vi "Initialize.vi"(5 "plugin settings":T1[](array[typedef]), 7 "Components":refnum<class "Component.lvclass">[](array[class]), 8 "error in (no error)":errorcluster, 9 "Group Configurations":refnum<class "Group Configuration.lvclass">[](array[class]), 10 "Thread Configuration":refnum<class "Thread Configuration.lvclass">, 11 "Plugin Thread in":refnum<class "Plugin Thread.lvclass">) -> (0 "error out":errorcluster, 3 "Plugin Thread out":refnum<class "Plugin Thread.lvclass">)   [LabVIEW 2017, in "DSF Core.lvlib" / "Plugin Thread.lvclass"]
uses:
  Plugin Thread.lvclass
  Component/Component.lvclass
  Configuration/Base/Thread/Thread Configuration.lvclass
  Configuration/Base/Group/Group Configuration.lvclass
  Typedefs/DSF Settings Info.ctl
  Typedefs/DSF Version Info.ctl
  DSF Core.lvlib
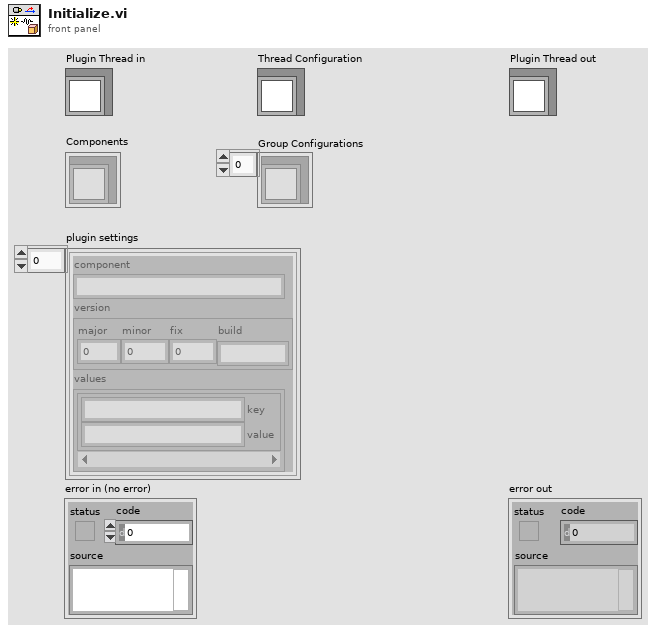
[diagram p1: front panel]
types:
  T1 = typedef "DSF Core.lvlib/DSF Settings Info.ctl" = cluster{"component":string, "version":T2, "values":cluster{"key":string, "value":string}[]}
  T2 = typedef "DSF Core.lvlib/DSF Version Info.ctl" = cluster{"major":u32, "minor":u32, "fix":u32, "build":string}
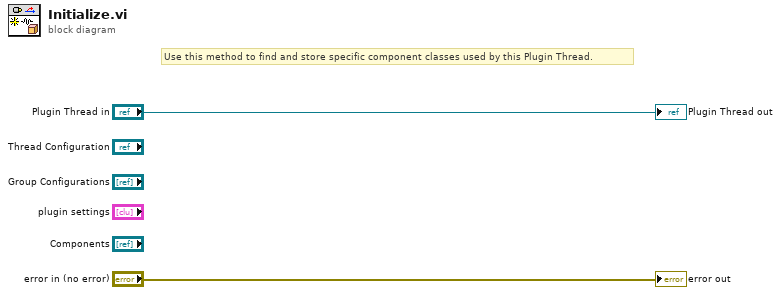
[diagram p0: block diagram]
diagram:
  # "Use this method to find and store specific component classes used by this Plugin Thread."
  "error out" <- "error in (no error)"
  "Plugin Thread out" <- "Plugin Thread in"
